vi "ToscaTTL-Wait For Condition.vi"(0 "When":string, 2 "Control Queue":refnum<queue>, 7 "Value":dbl, 11 "error in (no error)":errorcluster) -> (8 "trigger":bool, 15 "error out":errorcluster)   [LabVIEW 2020]
uses:
  Control Classes/Base Class/TTLController.lvclass
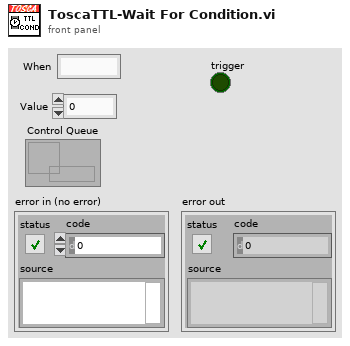
[diagram p1: front panel]
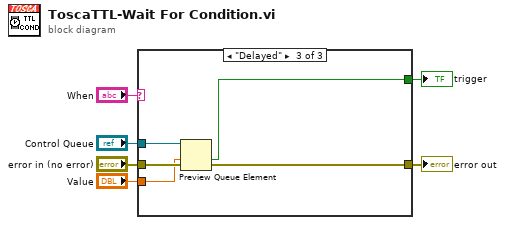
[diagram p0: block diagram]
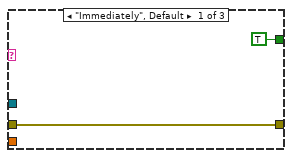
[diagram p2: hidden frame]
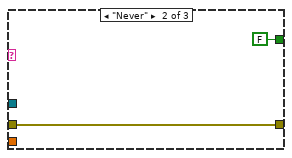
[diagram p3: hidden frame]
diagram:
  n1 = case shown="\"Delayed\"" "When" {
    tunnel: "error in (no error)" -> [w8 w10 w14]
    tunnel: [w8 w10 w14] -> w5
    tunnel: "Control Queue" -> [_ _ w13]
    tunnel: [TRUE FALSE w12] -> w3
    tunnel: "Value" -> [_ _ w11]
    frame "Immediately", Default {
    }
    frame "Never" {
    }
    frame "Delayed" {
      n2 = Preview Queue Element(queue=w13, timeout in ms (-1)=w11) -> (timed out?=w12:bool)  [unwired: 1 in, 3 out]
    }
  }
  "error out" <- w5
  "trigger" <- w3
